vi "Set Camera Configuration.vi"(8 "error in (no error)":errorcluster, 11 "CCDCamera in":refnum<class "CCDCamera.lvclass">) -> (0 "error out":errorcluster, 3 "CCDCamera out":refnum<class "CCDCamera.lvclass">)   [LabVIEW 2018, in "CCDCamera.lvclass"]
doc: "Set the camera configuration\n\nThis function records the given operating parameters in the camera. However, the parameters will only bewritten if their last value is different from the most recent one."
uses:
  CCDCamera.lvclass
  C:/Users/observer/Desktop/SPARC4_ACS/SPARC4_ACS/Simulated_CCD_Camera/Simulated_CCD_Camera.lvclass
  Simulated_CCD_Camera/Simulated_CCD_Camera.lvclass
panel:
  out "x != y? 2":T1
  out "x != y?":T2
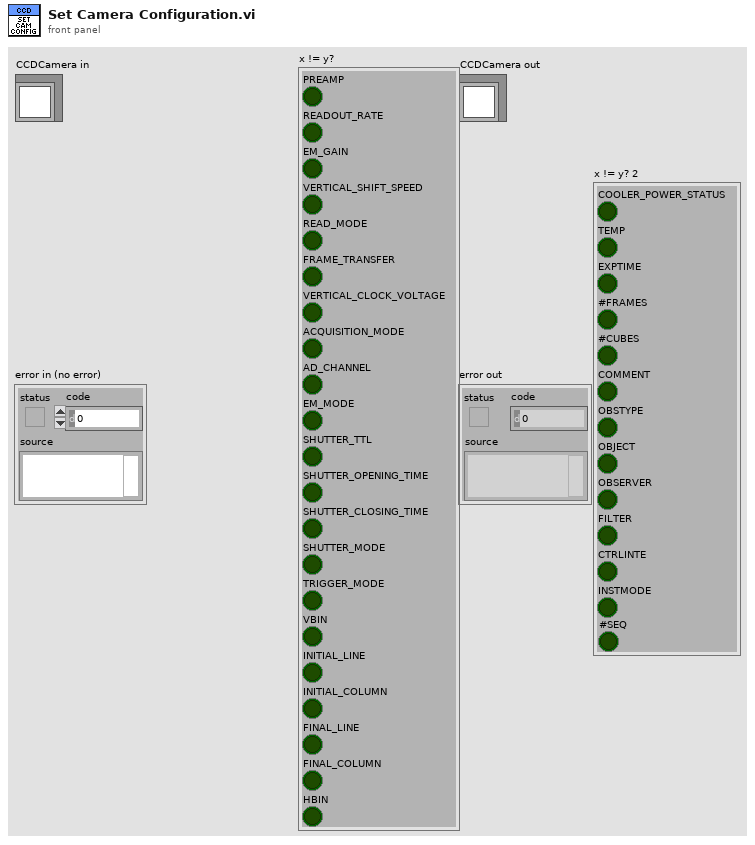
[diagram p1: front panel]
types:
  T1 = cluster{"COOLER_POWER_STATUS":bool, "TEMP":bool, "EXPTIME":bool, "#FRAMES":bool, "#CUBES":bool, "COMMENT":bool, "OBSTYPE":bool, "OBJECT":bool, "OBSERVER":bool, "FILTER":bool, "CTRLINTE":bool, "INSTMODE":bool, "#SEQ":bool}
  T2 = cluster{"PREAMP":bool, "READOUT_RATE":bool, "EM_GAIN":bool, "VERTICAL_SHIFT_SPEED":bool, "READ_MODE":bool, "FRAME_TRANSFER":bool, "VERTICAL_CLOCK_VOLTAGE":bool, "ACQUISITION_MODE":bool, "AD_CHANNEL":bool, "EM_MODE":bool, "SHUTTER_TTL":bool, "SHUTTER_OPENING_TIME":bool, "SHUTTER_CLOSING_TIME":bool, "SHUTTER_MODE":bool, "TRIGGER_MODE":bool, "VBIN":bool, "INITIAL_LINE":bool, "INITIAL_COLUMN":bool, "FINAL_LINE":bool, "FINAL_COLUMN":bool, "HBIN":bool}
  T3 = cluster{"PREAMP":u16, "READOUT_RATE":u16, "EM_GAIN":u16, "VERTICAL_SHIFT_SPEED":u16, "READ_MODE":u16, "FRAME_TRANSFER":bool, "VERTICAL_CLOCK_VOLTAGE":u16, "ACQUISITION_MODE":u16, "AD_CHANNEL":u16, "EM_MODE":u16, "SHUTTER_TTL":u16, "SHUTTER_OPENING_TIME":u16, "SHUTTER_CLOSING_TIME":u16, "SHUTTER_MODE":u16, "TRIGGER_MODE":u16, "VBIN":u16, "INITIAL_LINE":u16, "INITIAL_COLUMN":u16, "FINAL_LINE":u16, "FINAL_COLUMN":u16, "HBIN":u16}
  T4 = cluster{"COOLER_POWER_STATUS":u16, "TEMP":i32, "EXPTIME":dbl, "#FRAMES":u32, "#CUBES":u32, "COMMENT":string, "OBSTYPE":string, "OBJECT":string, "OBSERVER":string, "FILTER":string, "CTRLINTE":string, "INSTMODE":string, "#SEQ":u32}
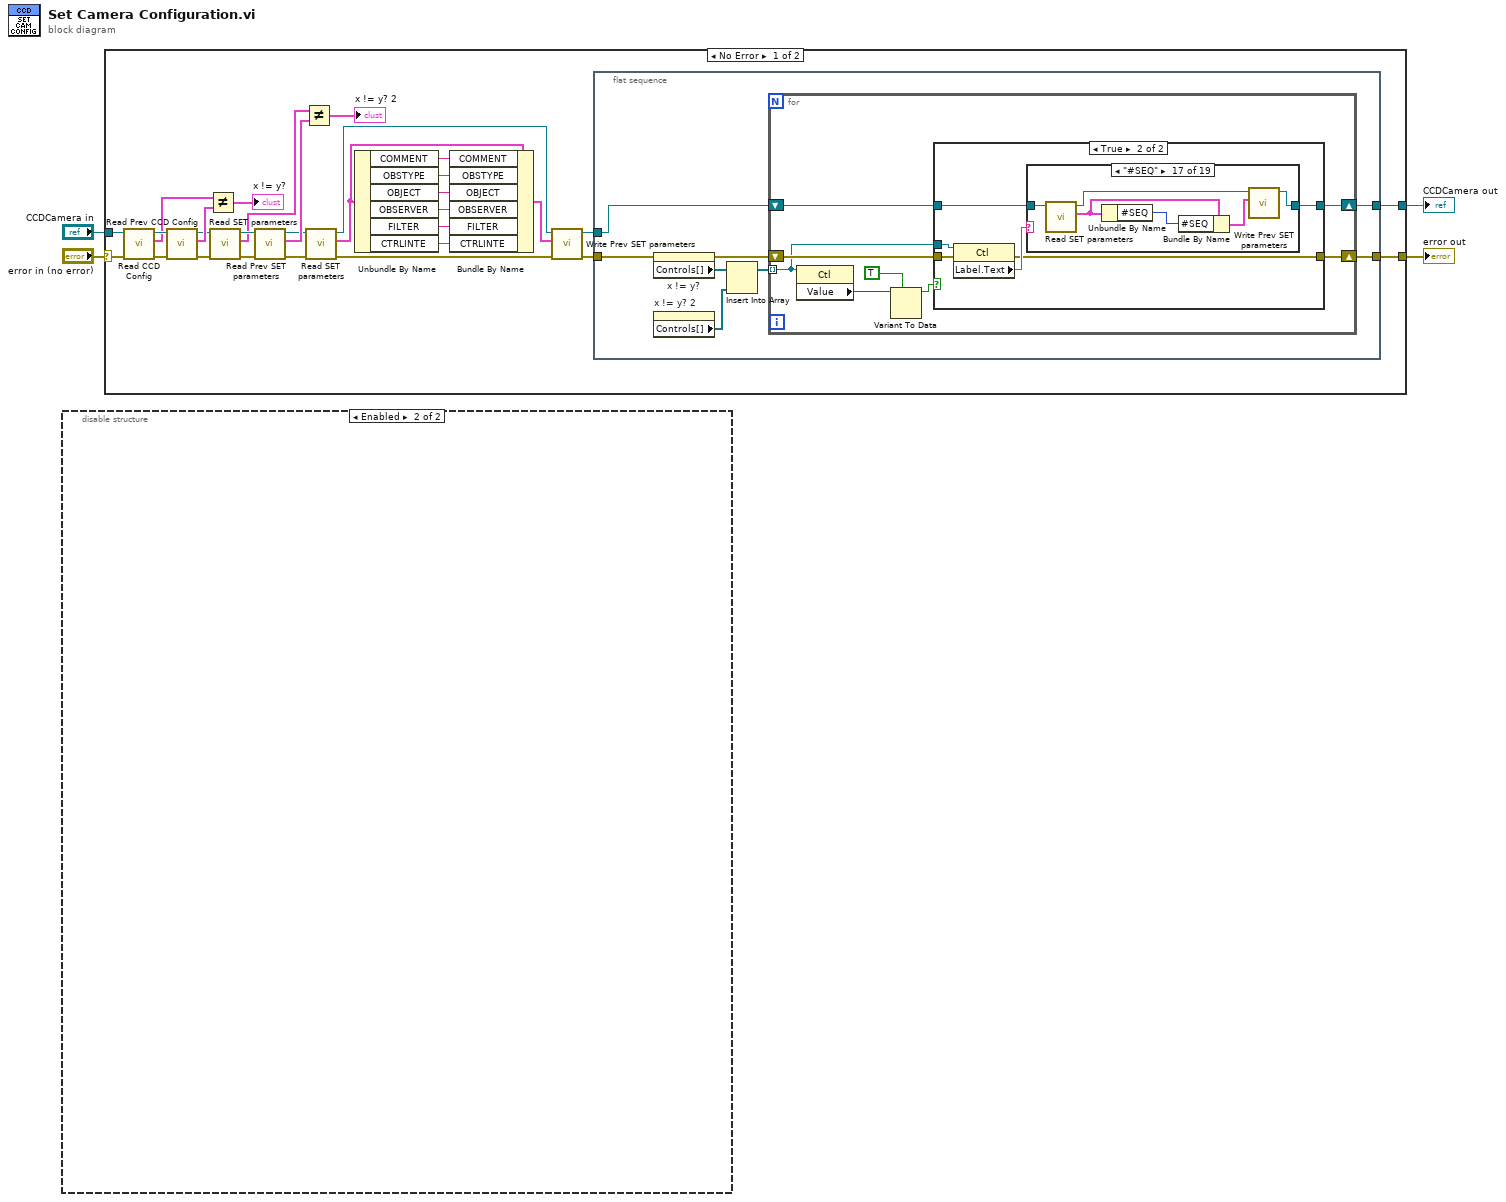
[diagram p0: block diagram]
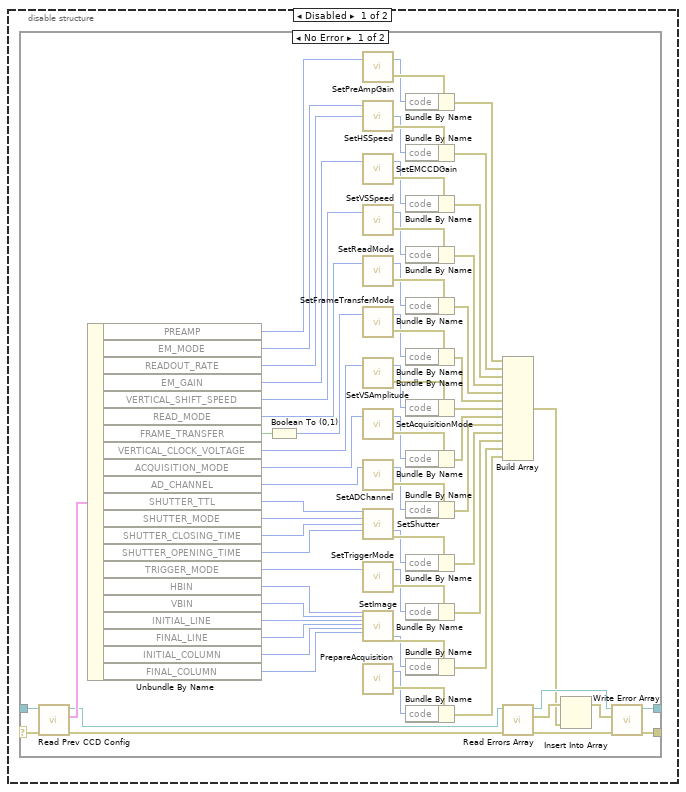
[diagram p2: hidden frame]
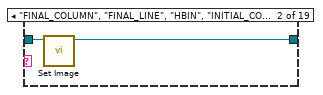
[diagram p6: hidden frame]
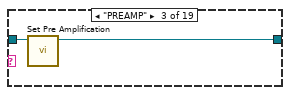
[diagram p7: hidden frame]
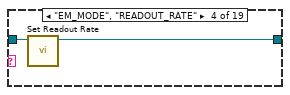
[diagram p8: hidden frame]
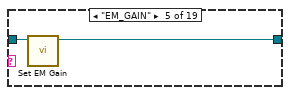
[diagram p9: hidden frame]
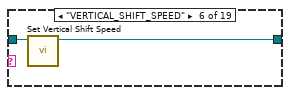
[diagram p10: hidden frame]
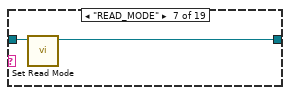
[diagram p11: hidden frame]
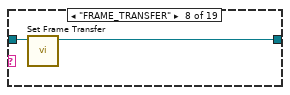
[diagram p12: hidden frame]
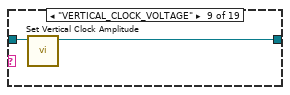
[diagram p13: hidden frame]
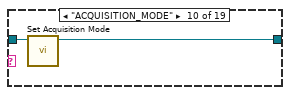
[diagram p14: hidden frame]
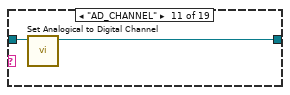
[diagram p15: hidden frame]
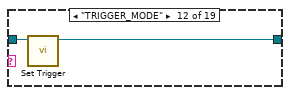
[diagram p16: hidden frame]
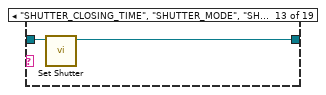
[diagram p17: hidden frame]
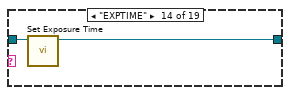
[diagram p18: hidden frame]
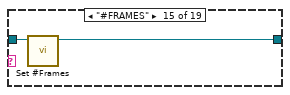
[diagram p19: hidden frame]
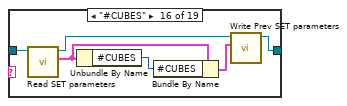
[diagram p20: hidden frame]
diagram:
  n1 = disable-structure shown="Enabled" {
    frame Disabled {
      n2 = case shown="No Error" {
        selector: _ -> [w77 w79]
        tunnel: [w52 w79] -> _
        tunnel: [w53 w78] -> _
        tunnel: _ -> [w51 w78]
        frame No Error {
          n3 = call-dynamic "Read Prev CCD Config.vi"("error in (no error)"=w77, "Simulated_CCD_Camera in"=w51) -> ("error out"=w11:errorcluster, "Prev CCD Config"=w76:T3, "Simulated_CCD_Camera out"=w9:refnum<class "CCDCamera.lvclass">)  [unwired: 7 in]
          n4 = Unbundle By Name(w76) -> ("PREAMP"=w75:u16, "EM_MODE"=w74:u16, "READOUT_RATE"=w73:u16, "EM_GAIN"=w72:u16, "VERTICAL_SHIFT_SPEED"=w71:u16, "READ_MODE"=w70:u16, "FRAME_TRANSFER"=w68:bool, "VERTICAL_CLOCK_VOLTAGE"=w67:u16, "ACQUISITION_MODE"=w66:u16, "AD_CHANNEL"=w65:u16, "SHUTTER_TTL"=w64:u16, "SHUTTER_MODE"=w63:u16, "SHUTTER_CLOSING_TIME"=w62:u16, "SHUTTER_OPENING_TIME"=w61:u16, "TRIGGER_MODE"=w60:u16, "HBIN"=w59:u16, "VBIN"=w58:u16, "INITIAL_LINE"=w57:u16, "FINAL_LINE"=w56:u16, "INITIAL_COLUMN"=w55:u16, "FINAL_COLUMN"=w54:u16)
          n5 = Boolean To (0,1)(Boolean=w68) -> (0, 1=w69:i16)
          n6 = call <userlib>:"SetPreAmpGain.vi"("index"=w75) -> ("error out"=w50:errorcluster, "DLL error code"=w49:u32)  [unwired: 1 in]
          n7 = call <userlib>:"SetHSSpeed.vi"("index"=w73, "type"=w74) -> ("error out"=w47:errorcluster, "DLL error code"=w46:u32)  [unwired: 2 in]
          n8 = call <userlib>:"SetEMCCDGain.vi"("gain"=w72) -> ("error out"=w44:errorcluster, "DLL error code"=w43:u32)  [unwired: 1 in]
          n9 = call <userlib>:"SetVSSpeed.vi"("index"=w71) -> ("error out"=w41:errorcluster, "DLL error code"=w40:u32)  [unwired: 1 in]
          n10 = call <userlib>:"SetReadMode.vi"("mode"=w70) -> ("error out"=w38:errorcluster, "DLL error code"=w37:u32)  [unwired: 1 in]
          n11 = call <userlib>:"SetFrameTransferMode.vi"("mode"=w69) -> ("error out"=w35:errorcluster, "DLL error code"=w34:u32)  [unwired: 1 in]
          n12 = call <userlib>:"SetVSAmplitude.vi"("amplitude"=w67) -> ("error out"=w32:errorcluster, "DLL error code"=w31:u32)  [unwired: 1 in]
          n13 = call <userlib>:"SetAcquisitionMode.vi"("mode"=w66) -> ("error out"=w16:errorcluster, "DLL error code"=w15:u32)  [unwired: 1 in]
          n14 = call <userlib>:"SetADChannel.vi"("channel"=w65) -> ("error out"=w29:errorcluster, "DLL error code"=w28:u32)  [unwired: 1 in]
          n15 = call <userlib>:"SetShutter.vi"("type"=w64, "mode"=w63, "closingtime"=w62, "openingtime"=w61) -> ("DLL error code"=w13:u32, "error out"=w14:errorcluster)  [unwired: 10 in]
          n16 = call <userlib>:"SetTriggerMode.vi"("mode"=w60) -> ("error out"=w26:errorcluster, "DLL error code"=w25:u32)  [unwired: 1 in]
          n17 = call <userlib>:"SetImage.vi"("hbin"=w59, "vbin"=w58, "hstart"=w57, "hend"=w56, "vstart"=w55, "vend"=w54) -> ("DLL error code"=w22:u32, "error out"=w23:errorcluster)  [unwired: 20 in]
          n18 = call <userlib>:"PrepareAcquisition.vi"() -> ("error out"=w20:errorcluster, "DLL error code"=w19:u32)  [unwired: 2 in]
          n19 = Bundle By Name(cluster=w50, "code"=w49) -> (w48:errorcluster)
          n20 = Bundle By Name(cluster=w47, "code"=w46) -> (w45:errorcluster)
          n21 = Bundle By Name(cluster=w44, "code"=w43) -> (w42:errorcluster)
          n22 = Bundle By Name(cluster=w41, "code"=w40) -> (w39:errorcluster)
          n23 = Bundle By Name(cluster=w38, "code"=w37) -> (w36:errorcluster)
          n24 = Bundle By Name(cluster=w35, "code"=w34) -> (w33:errorcluster)
          n25 = Bundle By Name(cluster=w32, "code"=w31) -> (w30:errorcluster)
          n26 = Bundle By Name(cluster=w16, "code"=w15) -> (w17:errorcluster)
          n27 = Bundle By Name(cluster=w29, "code"=w28) -> (w27:errorcluster)
          n28 = Bundle By Name(cluster=w14, "code"=w13) -> (w12:errorcluster)
          n29 = Bundle By Name(cluster=w26, "code"=w25) -> (w24:errorcluster)
          n30 = Bundle By Name(cluster=w23, "code"=w22) -> (w21:errorcluster)
          n31 = Bundle By Name(cluster=w20, "code"=w19) -> (w18:errorcluster)
          n32 = Build Array(w48, w45, w42, w39, w36, w33, w30, w17, w27, w12, w24, w21, w18) -> (w5:errorcluster[])
          n33 = call "Read Errors Array.vi"("error in (no error)"=w11, "Simulated_CCD_Camera in"=w9) -> ("error out"=w10:errorcluster, "Errors array"=w7:errorcluster[], "Simulated_CCD_Camera out"=w8:refnum<class "CCDCamera.lvclass">)  [unwired: 7 in]
          n34 = Insert Into Array(array=w7, new element=w5) -> (w6:errorcluster[])  [unwired: 1 in]
          n35 = call "Write Error Array.vi"("error in (no error)"=w10, "Errors array"=w6, "Simulated_CCD_Camera in"=w8) -> ("error out"=w52:errorcluster, "Simulated_CCD_Camera out"=w53:refnum<class "CCDCamera.lvclass">)  [unwired: 7 in]
        }
        frame Error {
        }
      }
    }
    frame Enabled {
    }
  }
  n36 = case shown="No Error" "error in (no error)" {
    selector: "error in (no error)" -> [w108 w180]
    tunnel: [w107 w180] -> w4
    tunnel: [w106 w179] -> w3
    tunnel: "CCDCamera in" -> [w105 w179]
    frame No Error {
      n37 = call "Read CCD Config.vi"("error in (no error)"=w108, "CCDCamera in"=w105) -> ("error out"=w102:errorcluster, "CCD Config"=w98:T3, "CCDCamera out"=w103:refnum<class "CCDCamera.lvclass">)  [unwired: 7 in]
      n38 = call-dynamic "Read Prev CCD Config.vi"("error in (no error)"=w102, "Simulated_CCD_Camera in"=w103) -> ("error out"=w95:errorcluster, "Prev CCD Config"=w104:T3, "Simulated_CCD_Camera out"=w96:refnum<class "CCDCamera.lvclass">)  [unwired: 7 in]
      n39 = Not Equal?(x=w98, y=w104) -> (x != y?=→"x != y?":T2)
      n40 = call-dynamic "Read SET parameters.vi"("error in (no error)"=w95, "Simulated_CCD_Camera in"=w96) -> ("error out"=w101:errorcluster, "New SET parameters"=w97:T4, "Simulated_CCD_Camera out"=w100:refnum<class "CCDCamera.lvclass">)  [unwired: 7 in]
      n41 = call-dynamic "Read Prev SET parameters.vi"("error in (no error)"=w101, "Simulated_CCD_Camera in"=w100) -> ("error out"=w89:errorcluster, "Old SET parameters"=w99:T4, "Simulated_CCD_Camera out"=w90:refnum<class "CCDCamera.lvclass">)  [unwired: 7 in]
      n42 = Not Equal?(x=w97, y=w99) -> (x != y?=→"x != y? 2":T1)
      n43 = call-dynamic "Read SET parameters.vi"("error in (no error)"=w89, "Simulated_CCD_Camera in"=w90) -> ("error out"=w82:errorcluster, "New SET parameters"=w93:T4, "Simulated_CCD_Camera out"=w94:refnum<class "CCDCamera.lvclass">)  [unwired: 7 in]
      n44 = Unbundle By Name(w93) -> ("COMMENT"=w91:string, "OBSTYPE"=w83:string, "OBJECT"=w84:string, "OBSERVER"=w85:string, "FILTER"=w86:string, "CTRLINTE"=w81:string)
      n45 = Bundle By Name(cluster=w93, "COMMENT"=w91, "OBSTYPE"=w83, "OBJECT"=w84, "OBSERVER"=w85, "FILTER"=w86, "CTRLINTE"=w81) -> (w92:T4)
      n46 = call-dynamic "Write Prev SET parameters.vi"("error in (no error)"=w82, "Old SET parameters"=w92, "Simulated_CCD_Camera in"=w94) -> ("error out"=w87:errorcluster, "Simulated_CCD_Camera out"=w88:refnum<class "CCDCamera.lvclass">)  [unwired: 7 in]
      n47 = flat-sequence {
        tunnel: w87 -> [w111]
        tunnel: [w117] -> w107
        tunnel: w88 -> [w115]
        tunnel: [w114] -> w106
        frame #0 {
          n48 = property on="x != y?" class="Clust (strict)"(error in=w111) -> (error out=w116:errorcluster, "Controls[]"=w113:refnum<vi>[])  [unwired: 1 in, 1 out]
          n49 = property on="x != y? 2" class="Clust (strict)"() -> ("Controls[]"=w110:refnum<vi>[])  [unwired: 2 in, 2 out]
          n50 = Insert Into Array(array=w113, new element=w110) -> (w112:refnum<vi>[])  [unwired: 1 in]
          n51 = for {
            tunnel: w112 -> [w124] mode=indexing
            shift-right: [w118] -> w117
            shift-left: w116 -> [w125]
            shift-right: [w119] -> w114
            shift-left: w115 -> [w120]
            n52 = property class="Ctl"(reference=w124) -> ("Value"=w123:variant)  [unwired: 1 in, 2 out]
            n53 = Variant To Data(type=TRUE, Variant=w123) -> (data=w121:bool)  [unwired: 1 in, 1 out]
            n54 = case shown="True" w121 {
              tunnel: w124 -> [_ w133]
              tunnel: [w127 w128] -> w118
              tunnel: w125 -> [w127 w131]
              tunnel: w120 -> [w126 w130]
              tunnel: [w126 w129] -> w119
              frame False {
              }
              frame True {
                n55 = property class="Ctl"(reference=w133, error in=w131) -> (error out=w128:errorcluster, "Label.Text"=w132:string)  [unwired: 1 out]
                n56 = case shown="\"#SEQ\"" w132 {
                  tunnel: w130 -> [w134 w136 w138 w139 w142 w144 w146 w148 w149 w152 w154 w155 w158 w160 w161 w168 w174 w175 w178]
                  tunnel: [w134 w135 w137 w140 w141 w143 w145 w147 w150 w151 w153 w156 w157 w159 w162 w167 w173 w176 w177] -> w129
                  frame "False", Default {
                  }
                  frame "FINAL_COLUMN", "FINAL_LINE", "HBIN", "INITIAL_COLUMN", "INITIAL_LINE", "VBIN" {
                    n57 = call-dynamic "Set Image.vi"("CCDCamera in"=w136) -> ("CCDCamera out"=w135:refnum<class "CCDCamera.lvclass">)  [unwired: 9 in, 1 out]
                  }
                  frame "PREAMP" {
                    n58 = call-dynamic "Set Pre Amplification.vi"("CCDCamera in"=w138) -> ("CCDCamera out"=w137:refnum<class "CCDCamera.lvclass">)  [unwired: 9 in, 1 out]
                  }
                  frame "EM_MODE", "READOUT_RATE" {
                    n59 = call-dynamic "Set Readout Rate.vi"("CCDCamera in"=w139) -> ("CCDCamera out"=w140:refnum<class "CCDCamera.lvclass">)  [unwired: 9 in, 1 out]
                  }
                  frame "EM_GAIN" {
                    n60 = call-dynamic "Set EM Gain.vi"("CCDCamera in"=w142) -> ("CCDCamera out"=w141:refnum<class "CCDCamera.lvclass">)  [unwired: 9 in, 1 out]
                  }
                  frame "VERTICAL_SHIFT_SPEED" {
                    n61 = call-dynamic "Set Vertical Shift Speed.vi"("CCDCamera in"=w144) -> ("CCDCamera out"=w143:refnum<class "CCDCamera.lvclass">)  [unwired: 9 in, 1 out]
                  }
                  frame "READ_MODE" {
                    n62 = call-dynamic "Set Read Mode.vi"("CCDCamera in"=w146) -> ("CCDCamera out"=w145:refnum<class "CCDCamera.lvclass">)  [unwired: 9 in, 1 out]
                  }
                  frame "FRAME_TRANSFER" {
                    n63 = call-dynamic "Set Frame Transfer.vi"("CCDCamera in"=w148) -> ("CCDCamera out"=w147:refnum<class "CCDCamera.lvclass">)  [unwired: 9 in, 1 out]
                  }
                  frame "VERTICAL_CLOCK_VOLTAGE" {
                    n64 = call-dynamic "Set Vertical Clock Amplitude.vi"("CCDCamera in"=w149) -> ("CCDCamera out"=w150:refnum<class "CCDCamera.lvclass">)  [unwired: 9 in, 1 out]
                  }
                  frame "ACQUISITION_MODE" {
                    n65 = call-dynamic "Set Acquisition Mode.vi"("CCDCamera in"=w152) -> ("CCDCamera out"=w151:refnum<class "CCDCamera.lvclass">)  [unwired: 9 in, 1 out]
                  }
                  frame "AD_CHANNEL" {
                    n66 = call-dynamic "Set Analogical to Digital Channel.vi"("CCDCamera in"=w154) -> ("CCDCamera out"=w153:refnum<class "CCDCamera.lvclass">)  [unwired: 9 in, 1 out]
                  }
                  frame "TRIGGER_MODE" {
                    n67 = call-dynamic "Set Trigger.vi"("CCDCamera in"=w155) -> ("CCDCamera out"=w156:refnum<class "CCDCamera.lvclass">)  [unwired: 9 in, 1 out]
                  }
                  frame "SHUTTER_CLOSING_TIME", "SHUTTER_MODE", "SHUTTER_OPENING_TIME", "SHUTTER_TTL" {
                    n68 = call-dynamic "Set Shutter.vi"("CCDCamera in"=w158) -> ("CCDCamera out"=w157:refnum<class "CCDCamera.lvclass">)  [unwired: 9 in, 1 out]
                  }
                  frame "EXPTIME" {
                    n69 = call-dynamic "Set Exposure Time.vi"("CCDCamera in"=w160) -> ("CCDCamera out"=w159:refnum<class "CCDCamera.lvclass">)  [unwired: 9 in, 1 out]
                  }
                  frame "#FRAMES" {
                    n70 = call-dynamic "Set #Frames.vi"("CCDCamera in"=w161) -> ("CCDCamera out"=w162:refnum<class "CCDCamera.lvclass">)  [unwired: 9 in, 1 out]
                  }
                  frame "#CUBES" {
                    n71 = call-dynamic "Read SET parameters.vi"("Simulated_CCD_Camera in"=w168) -> ("New SET parameters"=w165:T4, "Simulated_CCD_Camera out"=w166:refnum<class "CCDCamera.lvclass">)  [unwired: 8 in, 1 out]
                    n72 = Unbundle By Name(w165) -> ("#CUBES"=w164:u32)
                    n73 = Bundle By Name(cluster=w165, "#CUBES"=w164) -> (w163:T4)
                    n74 = call-dynamic "Write Prev SET parameters.vi"("Old SET parameters"=w163, "Simulated_CCD_Camera in"=w166) -> ("Simulated_CCD_Camera out"=w167:refnum<class "CCDCamera.lvclass">)  [unwired: 8 in, 1 out]
                  }
                  frame "#SEQ" {
                    n75 = call-dynamic "Read SET parameters.vi"("Simulated_CCD_Camera in"=w174) -> ("New SET parameters"=w171:T4, "Simulated_CCD_Camera out"=w172:refnum<class "CCDCamera.lvclass">)  [unwired: 8 in, 1 out]
                    n76 = Unbundle By Name(w171) -> ("#SEQ"=w170:u32)
                    n77 = Bundle By Name(cluster=w171, "#SEQ"=w170) -> (w169:T4)
                    n78 = call-dynamic "Write Prev SET parameters.vi"("Old SET parameters"=w169, "Simulated_CCD_Camera in"=w172) -> ("Simulated_CCD_Camera out"=w173:refnum<class "CCDCamera.lvclass">)  [unwired: 8 in, 1 out]
                  }
                  frame "COOLER_POWER_STATUS" {
                    n79 = call-dynamic "Set Cooler Power Status.vi"("CCDCamera in"=w175) -> ("CCDCamera out"=w176:refnum<class "CCDCamera.lvclass">)  [unwired: 9 in, 1 out]
                  }
                  frame "TEMP" {
                    n80 = call-dynamic "Set Temperature.vi"("CCDCamera in"=w178) -> ("CCDCamera out"=w177:refnum<class "CCDCamera.lvclass">)  [unwired: 9 in, 1 out]
                  }
                }
              }
            }
          }
        }
      }
    }
    frame Error {
    }
  }
  "error out" <- w4
  "CCDCamera out" <- w3
